vi "nanocal -- nuclear schottky fit -- 2x2 -- V9.vi"() -> ()   [LabVIEW 2021] (continued)
\"Imoff\" -> 0.000000000000   ,  \"στ1\" -> 0.000000000000   ,  \"στS\" -> 0.000000000000   ,  \"στN\" -> 0.000000000000    |>   , \r\"IDS0389_210910_RAW_cal__ref_\" ->   <|    \"ζ\" -> 0.019465629154   ,  \"τ1\" -> 0.035571135590   ,  \"τS\" -> 0.015266533820   ,  \"τN\" -> 0.000260285661   ,  \"τC\" -> 0.004529981538   ,  \"κ0\" -> 0.000000010200   ,  \"mm1\" -> 0.000067219896   ,  \"mm2\" -> 0.019697516293   ,  \"mm3\" -> 0.036165439730   ,  \"T\" -> 1.520000000000   ,  \"B\" -> 8.000000000000   ,  \"θ\" -> 0.000000000000   ,  \"Reoff\" -> -551020.408163265324   ,  \"Imoff\" -> 0.000000000000   ,  \"στ1\" -> 0.011471207658   ,  \"στS\" -> 0.000401132713   ,  \"στN\" -> 0.000048991456    |>   , \r\"IDS0389_210910_RAW_cal__sam_\" ->   <|    \"ζ\" -> 0.011148198813   ,  \"τ1\" -> 0.038849151842   ,  \"τS\" -> 0.019213865355   ,  \"τN\" -> 0.000045035153   ,  \"τC\" -> 0.005536708133   ,  \"κ0\" -> 0.000000011229   ,  \"mm1\" -> 0.000047596165   ,  \"mm2\" -> 0.024836509281   ,  \"mm3\" -> 0.038975357089   ,  \"T\" -> 1.520000000000   ,  \"B\" -> 8.000000000000   ,  \"θ\" -> 0.000000000000   ,  \"Reoff\" -> 0.000000000000   ,  \"Imoff\" -> 0.000000000000   ,  \"στ1\" -> 0.000000000000   ,  \"στS\" -> 0.000000000000   ,  \"στN\" -> 0.000000000000    |>   , \r\"IDS0390_210910_RAW_cal__ref_\" ->   <|    \"ζ\" -> 0.016838578105   ,  \"τ1\" -> 0.032747492196   ,  \"τS\" -> 0.011207679404   ,  \"τN\" -> 0.000117854318   ,  \"τC\" -> 0.003479559601   ,  \"κ0\" -> 0.000000013000   ,  \"mm1\" -> 0.000044274477   ,  \"mm2\" -> 0.014733756508   ,  \"mm3\" -> 0.032965260417   ,  \"T\" -> 1.900000000000   ,  \"B\" -> 8.000000000000   ,  \"θ\" -> 0.000000000000   ,  \"Reoff\" -> -346938.775510204024   ,  \"Imoff\" -> 0.000000000000   ,  \"στ1\" -> 0.005723858997   ,  \"στS\" -> 0.000088565552   ,  \"στN\" -> 0.000007225901    |>   , \r\"IDS0390_210910_RAW_cal__sam_\" ->   <|    \"ζ\" -> 0.010826949430   ,  \"τ1\" -> 0.038768037521   ,  \"τS\" -> 0.012925317198   ,  \"τN\" -> 0.000029157336   ,  \"τC\" -> 0.005196063884   ,  \"κ0\" -> 0.000000013864   ,  \"mm1\" -> 0.000039906108   ,  \"mm2\" -> 0.018195372076   ,  \"mm3\" -> 0.038823555195   ,  \"T\" -> 1.900000000000   ,  \"B\" -> 8.000000000000   ,  \"θ\" -> 0.000000000000   ,  \"Reoff\" -> 0.000000000000   ,  \"Imoff\" -> 0.000000000000   ,  \"στ1\" -> 0.000000000000   ,  \"στS\" -> 0.000000000000   ,  \"στN\" -> 0.000000000000    |>   , \r\"IDS0391_210910_RAW_cal__ref_\" ->   <|    \"ζ\" -> 0.014193901830   ,  \"τ1\" -> 0.092879337404   ,  \"τS\" -> 0.043047307828   ,  \"τN\" -> 0.000265545099   ,  \"τC\" -> 0.003595748456   ,  \"κ0\" -> 0.000000008330   ,  \"mm1\" -> 0.000046539933   ,  \"mm2\" -> 0.046932456699   ,  \"mm3\" -> 0.093423720537   ,  \"T\" -> 1.250000000000   ,  \"B\" -> 8.000000000000   ,  \"θ\" -> 0.000000000000   ,  \"Reoff\" -> -224489.795918366871   ,  \"Imoff\" -> 0.000000000000   ,  \"στ1\" -> 0.004842916086   ,  \"στS\" -> 0.000245036767   ,  \"στN\" -> 0.000003156227    |>   , \r\"IDS0391_210910_RAW_cal__sam_\" ->   <|    \"ζ\" -> 0.010962610928   ,  \"τ1\" -> 0.040398807374   ,  \"τS\" -> 0.051328988590   ,  \"τN\" -> 0.000070281011   ,  \"τC\" -> 0.006422533164   ,  \"κ0\" -> 0.000000008958   ,  \"mm1\" -> 0.000062039854   ,  \"mm2\" -> 0.040240103995   ,  \"mm3\" -> 0.058481936484   ,  \"T\" -> 1.250000000000   ,  \"B\" -> 8.000000000000   ,  \"θ\" -> 0.000000000000   ,  \"Reoff\" -> 0.000000000000   ,  \"Imoff\" -> 0.000000000000   ,  \"στ1\" -> 0.000000000000   ,  \"στS\" -> 0.000000000000   ,  \"στN\" -> 0.000000000000    |>   , \r\"IDS0392_210910_RAW_cal__ref_\" ->   <|    \"ζ\" -> 0.015915665125   ,  \"τ1\" -> 0.061543395288   ,  \"τS\" -> 0.031670398058   ,  \"τN\" -> 0.000248131167   ,  \"τC\" -> 0.003886930831   ,  \"κ0\" -> 0.000000009270   ,  \"mm1\" -> 0.000054412441   ,  \"mm2\" -> 0.035659745539   ,  \"mm3\" -> 0.062142701987   ,  \"T\" -> 1.390000000000   ,  \"B\" -> 8.000000000000   ,  \"θ\" -> 0.000000000000   ,  \"Reoff\" -> -224489.795918366871   ,  \"Imoff\" -> 0.000000000000   ,  \"στ1\" -> 0.005114709163   ,  \"στS\" -> 0.000350050575   ,  \"στN\" -> 0.000004808789    |>   , \r\"IDS0392_210910_RAW_cal__sam_\" ->   <|    \"ζ\" -> 0.010962610928   ,  \"τ1\" -> 0.040398807374   ,  \"τS\" -> 0.051328988590   ,  \"τN\" -> 0.000070281011   ,  \"τC\" -> 0.006422533164   ,  \"κ0\" -> 0.000000008958   ,  \"mm1\" -> 0.000062039854   ,  \"mm2\" -> 0.040240103995   ,  \"mm3\" -> 0.058481936484   ,  \"T\" -> 1.390000000000   ,  \"B\" -> 8.000000000000   ,  \"θ\" -> 0.000000000000   ,  \"Reoff\" -> 0.000000000000   ,  \"Imoff\" -> 0.000000000000   ,  \"στ1\" -> 0.000000000000   ,  \"στS\" -> 0.000000000000   ,  \"στN\" -> 0.000000000000    |>   , \r\"IDS0393_210910_RAW_cal__ref_\" ->   <|    \"ζ\" -> 0.014955256266   ,  \"τ1\" -> 0.026332624911   ,  \"τS\" -> 0.008352670277   ,  \"τN\" -> 0.000164111809   ,  \"τC\" -> 0.002903513034   ,  \"κ0\" -> 0.000000023300   ,  \"mm1\" -> 0.000031957834   ,  \"mm2\" -> 0.011225492804   ,  \"mm3\" -> 0.026622840052   ,  \"T\" -> 3.110000000000   ,  \"B\" -> 8.000000000000   ,  \"θ\" -> 0.000000000000   ,  \"Reoff\" -> -183673.469387754798   ,  \"Imoff\" -> 0.000000000000   ,  \"στ1\" -> 0.001054663608   ,  \"στS\" -> 0.000052081378   ,  \"στN\" -> 0.000002015225    |>   , \r\"IDS0393_210910_RAW_cal__sam_\" ->   <|    \"ζ\" -> 0.010962610928   ,  \"τ1\" -> 0.040398807374   ,  \"τS\" -> 0.051328988590   ,  \"τN\" -> 0.000070281011   ,  \"τC\" -> 0.006422533164   ,  \"κ0\" -> 0.000000008958   ,  \"mm1\" -> 0.000062039854   ,  \"mm2\" -> 0.040240103995   ,  \"mm3\" -> 0.058481936484   ,  \"T\" -> 3.110000000000   ,  \"B\" -> 8.000000000000   ,  \"θ\" -> 0.000000000000   ,  \"Reoff\" -> 0.000000000000   ,  \"Imoff\" -> 0.000000000000   ,  \"στ1\" -> 0.000000000000   ,  \"στS\" -> 0.000000000000   ,  \"στN\" -> 0.000000000000    |>   , \r\"IDS0394_210910_RAW_cal__ref_\" ->   <|    \"ζ\" -> 0.016050939839   ,  \"τ1\" -> 0.020478636674   ,  \"τS\" -> 0.005312059468   ,  \"τN\" -> 0.000195533635   ,  \"τC\" -> 0.002460552068   ,  \"κ0\" -> 0.000000057800   ,  \"mm1\" -> 0.000026789678   ,  \"mm2\" -> 0.007711278862   ,  \"mm3\" -> 0.020797115351   ,  \"T\" -> 5.750000000000   ,  \"B\" -> 8.000000000000   ,  \"θ\" -> 0.000000000000   ,  \"Reoff\" -> -61224.489795917645   ,  \"Imoff\" -> 0.000000000000   ,  \"στ1\" -> 0.004716029121   ,  \"στS\" -> 0.000047047015   ,  \"στN\" -> 0.000018531547    |>   , \r\"IDS0394_210910_RAW_cal__sam_\" ->   <|    \"ζ\" -> 0.010962610928   ,  \"τ1\" -> 0.040398807374   ,  \"τS\" -> 0.051328988590   ,  \"τN\" -> 0.000070281011   ,  \"τC\" -> 0.006422533164   ,  \"κ0\" -> 0.000000008958   ,  \"mm1\" -> 0.000062039854   ,  \"mm2\" -> 0.040240103995   ,  \"mm3\" -> 0.058481936484   ,  \"T\" -> 5.750000000000   ,  \"B\" -> 8.000000000000   ,  \"θ\" -> 0.000000000000   ,  \"Reoff\" -> 0.000000000000   ,  \"Imoff\" -> 0.000000000000   ,  \"στ1\" -> 0.000000000000   ,  \"στS\" -> 0.000000000000   ,  \"στN\" -> 0.000000000000    |>   , \r\"IDS0395_210910_RAW_cal__ref_\" ->   <|    \"ζ\" -> 0.014321636830   ,  \"τ1\" -> 0.097433211743   ,  \"τS\" -> 0.042062236733   ,  \"τN\" -> 0.000244628908   ,  \"τC\" -> 0.003645191846   ,  \"κ0\" -> 0.000000008580   ,  \"mm1\" -> 0.000047465439   ,  \"mm2\" -> 0.046040095215   ,  \"mm3\" -> 0.097903612141   ,  \"T\" -> 1.310000000000   ,  \"B\" -> 8.000000000000   ,  \"θ\" -> 0.000000000000   ,  \"Reoff\" -> -224489.795918366871   ,  \"Imoff\" -> 0.000000000000   ,  \"στ1\" -> 0.012889257014   ,  \"στS\" -> 0.000375170132   ,  \"στN\" -> 0.000004995458    |>   , \r\"IDS0395_210910_RAW_cal__sam_\" ->   <|    \"ζ\" -> 0.010962610928   ,  \"τ1\" -> 0.040398807374   ,  \"τS\" -> 0.051328988590   ,  \"τN\" -> 0.000070281011   ,  \"τC\" -> 0.006422533164   ,  \"κ0\" -> 0.000000008958   ,  \"mm1\" -> 0.000062039854   ,  \"mm2\" -> 0.040240103995   ,  \"mm3\" -> 0.058481936484   ,  \"T\" -> 1.310000000000   ,  \"B\" -> 8.000000000000   ,  \"θ\" -> 0.000000000000   ,  \"Reoff\" -> 0.000000000000   ,  \"Imoff\" -> 0.000000000000   ,  \"στ1\" -> 0.000000000000   ,  \"στS\" -> 0.000000000000   ,  \"στN\" -> 0.000000000000    |>   , \r\"IDS0407_220525_RAW_cal__ref_\" ->   <|    \"ζ\" -> 0.191981162244   ,  \"τ1\" -> 0.000715000000   ,  \"τS\" -> 0.013352458137   ,  \"τN\" -> 0.000004000000   ,  \"τC\" -> 0.002386991901   ,  \"κ0\" -> 0.000000000824   ,  \"mm1\" -> 0.000340641110   ,  \"mm2\" -> 0.000714825522   ,  \"mm3\" -> 0.017967171762   ,  \"T\" -> 0.200000000000   ,  \"B\" -> 0.000000000000   ,  \"θ\" -> 0.000000000000   ,  \"Reoff\" -> 7244897.959183672450   ,  \"Imoff\" -> 0.000000000000   ,  \"στ1\" -> 0.000308977102   ,  \"στS\" -> 0.004347578202   ,  \"στN\" -> 0.000003616273    |>   , \r\"IDS0407_220525_RAW_cal__sam_\" ->   <|    \"ζ\" -> 0.107728168967   ,  \"τ1\" -> 0.019656327090   ,  \"τS\" -> 0.016556579862   ,  \"τN\" -> 0.004758156992   ,  \"τC\" -> 0.001123654800   ,  \"κ0\" -> 0.000000000861   ,  \"mm1\" -> 0.000103510666   ,  \"mm2\" -> 0.011667063931   ,  \"mm3\" -> 0.032620341720   ,  \"T\" -> 0.200000000000   ,  \"B\" -> 0.000000000000   ,  \"θ\" -> 0.000000000000   ,  \"Reoff\" -> -36285714.285714283600   ,  \"Imoff\" -> 0.000000000000   ,  \"στ1\" -> 0.009912643228   ,  \"στS\" -> 0.001520300197   ,  \"στN\" -> 0.002063455636    |>   , \r\"IDS0408_220525_RAW_cal__ref_\" ->   <|    \"ζ\" -> 0.140207229242   ,  \"τ1\" -> 0.000100000000   ,  \"τS\" -> 0.011901792597   ,  \"τN\" -> 0.000001000000   ,  \"τC\" -> 0.001974879987   ,  \"κ0\" -> 0.000000001121   ,  \"mm1\" -> 0.000099990699   ,  \"mm2\" -> 0.000214969707   ,  \"mm3\" -> 0.015331569748   ,  \"T\" -> 0.250000000000   ,  \"B\" -> 0.000000000000   ,  \"θ\" -> 0.000000000000   ,  \"Reoff\" -> 571428.571428570895   ,  \"Imoff\" -> 0.000000000000   ,  \"στ1\" -> 0.000045284114   ,  \"στS\" -> 0.002476603384   ,  \"στN\" -> 0.000000665551    |>   , \r\"IDS0408_220525_RAW_cal__sam_\" ->   <|    \"ζ\" -> 0.086238207773   ,  \"τ1\" -> 0.018354133297   ,  \"τS\" -> 0.015001679768   ,  \"τN\" -> 0.004138272742   ,  \"τC\" -> 0.001377972360   ,  \"κ0\" -> 0.000000001190   ,  \"mm1\" -> 0.000101440698   ,  \"mm2\" -> 0.010941566515   ,  \"mm3\" -> 0.029479646155   ,  \"T\" -> 0.250000000000   ,  \"B\" -> 0.000000000000   ,  \"θ\" -> 0.000000000000   ,  \"Reoff\" -> -26000000.000000000000   ,  \"Imoff\" -> 0.000000000000   ,  \"στ1\" -> 0.004778614510   ,  \"στS\" -> 0.000718856892   ,  \"στN\" -> 0.001132000122    |>   , \r\"IDS0409_220525_RAW_cal__ref_\" ->   <|    \"ζ\" -> 0.126868069995   ,  \"τ1\" -> 0.000131000000   ,  \"τS\" -> 0.010549947054   ,  \"τN\" -> 0.000001000000   ,  \"τC\" -> 0.002473035290   ,  \"κ0\" -> 0.000000001433   ,  \"mm1\" -> 0.000130984950   ,  \"mm2\" -> 0.000234311726   ,  \"mm3\" -> 0.014128263958   ,  \"T\" -> 0.300000000000   ,  \"B\" -> 0.000000000000   ,  \"θ\" -> 0.000000000000   ,  \"Reoff\" -> -408163.265306122600   ,  \"Imoff\" -> 0.000000000000   ,  \"στ1\" -> 0.000026668297   ,  \"στS\" -> 0.002148216121   ,  \"στN\" -> 0.000000592429    |>   , \r\"IDS0409_220525_RAW_cal__sam_\" ->   <|    \"ζ\" -> 0.056561047780   ,  \"τ1\" -> 0.014299678758   ,  \"τS\" -> 0.013769239985   ,  \"τN\" -> 0.003071380883   ,  \"τC\" -> 0.001651608796   ,  \"κ0\" -> 0.000000001520   ,  \"mm1\" -> 0.000079784788   ,  \"mm2\" -> 0.009566648569   ,  \"mm3\" -> 0.024097998227   ,  \"T\" -> 0.300000000000   ,  \"B\" -> 0.000000000000   ,  \"θ\" -> 0.000000000000   ,  \"Reoff\" -> -9836734.693877555430   ,  \"Imoff\" -> 0.000000000000   ,  \"στ1\" -> 0.019869000982   ,  \"στS\" -> 0.002333902836   ,  \"στN\" -> 0.003131938876    |>   , \r\"IDS0410_220525_RAW_cal__ref_\" ->   <|    \"ζ\" -> 0.254310189332   ,  \"τ1\" -> 0.000715000000   ,  \"τS\" -> 0.015590963153   ,  \"τN\" -> 0.000004000000   ,  \"τC\" -> 0.001826387859   ,  \"κ0\" -> 0.000000000621   ,  \"mm1\" -> 0.000344204204   ,  \"mm2\" -> 0.000714835949   ,  \"mm3\" -> 0.021043268891   ,  \"T\" -> 0.170000000000   ,  \"B\" -> 0.000000000000   ,  \"θ\" -> 0.000000000000   ,  \"Reoff\" -> -38967346.938775509600   ,  \"Imoff\" -> 0.000000000000   ,  \"στ1\" -> 0.000454190024   ,  \"στS\" -> 0.005556659278   ,  \"στN\" -> 0.000004239490    |>   , \r\"IDS0410_220525_RAW_cal__sam_\" ->   <|    \"ζ\" -> 0.124885425459   ,  \"τ1\" -> 0.026966294273   ,  \"τS\" -> 0.017799663974   ,  \"τN\" -> 0.005835531331   ,  \"τC\" -> 0.001338388753   ,  \"κ0\" -> 0.000000000710   ,  \"mm1\" -> 0.000140185240   ,  \"mm2\" -> 0.014066781222   ,  \"mm3\" -> 0.040684603290   ,  \"T\" -> 0.170000000000   ,  \"B\" -> 0.000000000000   ,  \"θ\" -> 0.000000000000   ,  \"Reoff\" -> -36285714.285714283600   ,  \"Imoff\" -> 0.000000000000   ,  \"στ1\" -> 0.125291630718   ,  \"στS\" -> 0.008513087182   ,  \"στN\" -> 0.016544280517    |>   , \r\"IDS0411_220525_RAW_cal__ref_\" ->   <|    \"ζ\" -> 0.285546164030   ,  \"τ1\" -> 0.000715000000   ,  \"τS\" -> 0.017341393602   ,  \"τN\" -> 0.000004000000   ,  \"τC\" -> 0.001738862257   ,  \"κ0\" -> 0.000000000531   ,  \"mm1\" -> 0.000363792434   ,  \"mm2\" -> 0.000714850091   ,  \"mm3\" -> 0.023673523941   ,  \"T\" -> 0.150000000000   ,  \"B\" -> 0.000000000000   ,  \"θ\" -> 0.000000000000   ,  \"Reoff\" -> -60000000.000000000000   ,  \"Imoff\" -> 0.000000000000   ,  \"στ1\" -> 0.002198366616   ,  \"στS\" -> 0.030518183124   ,  \"στN\" -> 0.000021250478    |>   , \r\"IDS0411_220525_RAW_cal__sam_\" ->   <|    \"ζ\" -> 0.135609092663   ,  \"τ1\" -> 0.033619209304   ,  \"τS\" -> 0.020242350677   ,  \"τN\" -> 0.009065316224   ,  \"τC\" -> 0.001338388753   ,  \"κ0\" -> 0.000000000610   ,  \"mm1\" -> 0.000151964902   ,  \"mm2\" -> 0.015437467353   ,  \"mm3\" -> 0.052650218819   ,  \"T\" -> 0.150000000000   ,  \"B\" -> 0.000000000000   ,  \"θ\" -> 0.000000000000   ,  \"Reoff\" -> -36285714.285714283600   ,  \"Imoff\" -> 0.000000000000   ,  \"στ1\" -> 0.012006153279   ,  \"στS\" -> 0.002506054906   ,  \"στN\" -> 0.002275285607    |>   , \r\"IDS0412_220525_RAW_cal__ref_\" ->   <|    \"ζ\" -> 0.335616597388   ,  \"τ1\" -> 0.000100000000   ,  \"τS\" -> 0.019397772519   ,  \"τN\" -> 0.000001000000   ,  \"τC\" -> 0.001855570949   ,  \"κ0\" -> 0.000000000419   ,  \"mm1\" -> 0.000099994748   ,  \"mm2\" -> 0.000442151707   ,  \"mm3\" -> 0.027322747041   ,  \"T\" -> 0.120000000000   ,  \"B\" -> 0.000000000000   ,  \"θ\" -> 0.000000000000   ,  \"Reoff\" -> -114641566.265060246000   ,  \"Imoff\" -> 0.000000000000   ,  \"στ1\" -> 0.000060137518   ,  \"στS\" -> 0.005391505874   ,  \"στN\" -> 0.000000931452    |>   , \r\"IDS0412_220525_RAW_cal__sam_\" ->   <|    \"ζ\" -> 0.141872667412   ,  \"τ1\" -> 0.045522682755   ,  \"τS\" -> 0.024683404671   ,  \"τN\" -> 0.014187266741   ,  \"τC\" -> 0.001029575567   ,  \"κ0\" -> 0.000000000485   ,  \"mm1\" -> 0.000123931838   ,  \"mm2\" -> 0.018251391889   ,  \"mm3\" -> 0.072562291843   ,  \"T\" -> 0.120000000000   ,  \"B\" -> 0.000000000000   ,  \"θ\" -> 0.000000000000   ,  \"Reoff\" -> -36285714.285714283600   ,  \"Imoff\" -> 0.000000000000   ,  \"στ1\" -> 0.019575103663   ,  \"στS\" -> 0.006297786999   ,  \"στN\" -> 0.007663344539    |>   , \r\"IDS0413_220525_RAW_cal__ref_\" ->   <|    \"ζ\" -> 0.101522362019   ,  \"τ1\" -> 0.000131000000   ,  \"τS\" -> 0.009935467589   ,  \"τN\" -> 0.000001000000   ,  \"τC\" -> 0.002817089686   ,  \"κ0\" -> 0.000000001826   ,  \"mm1\" -> 0.000130982425   ,  \"mm2\" -> 0.000209693311   ,  \"mm3\" -> 0.013552655199   ,  \"T\" -> 0.360000000000   ,  \"B\" -> 0.000000000000   ,  \"θ\" -> 0.000000000000   ,  \"Reoff\" -> -346938.775510204024   ,  \"Imoff\" -> 0.000000000000   ,  \"στ1\" -> 0.000056432011   ,  \"στS\" -> 0.002135806697   ,  \"στN\" -> 0.000000647721    |>   , \r\"IDS0413_220525_RAW_cal__sam_\" ->   <|    \"ζ\" -> 0.044690907244   ,  \"τ1\" -> 0.013320614253   ,  \"τS\" -> 0.013760942515   ,  \"τN\" -> 0.002327045716   ,  \"τC\" -> 0.001523256988   ,  \"κ0\" -> 0.000000001960   ,  \"mm1\" -> 0.000059136229   ,  \"mm2\" -> 0.009591413737   ,  \"mm3\" -> 0.022000296296   ,  \"T\" -> 0.360000000000   ,  \"B\" -> 0.000000000000   ,  \"θ\" -> 0.000000000000   ,  \"Reoff\" -> -7142857.142857141800   ,  \"Imoff\" -> 0.000000000000   ,  \"στ1\" -> 0.002601583253   ,  \"στS\" -> 0.000378567326   ,  \"στN\" -> 0.000355149378    |>   , \r\"IDS0414_220525_RAW_cal__ref_\" ->   <|    \"ζ\" -> 0.086864800991   ,  \"τ1\" -> 0.000131000000   ,  \"τS\" -> 0.009397396069   ,  \"τN\" -> 0.000001000000   ,  \"τC\" -> 0.003391459878   ,  \"κ0\" -> 0.000000002303   ,  \"mm1\" -> 0.000130980131   ,  \"mm2\" -> 0.000206638483   ,  \"mm3\" -> 0.013399627137   ,  \"T\" -> 0.430000000000   ,  \"B\" -> 0.000000000000   ,  \"θ\" -> 0.000000000000   ,  \"Reoff\" -> -163265.306122449226   ,  \"Imoff\" -> 0.000000000000   ,  \"στ1\" -> 0.000060821776   ,  \"στS\" -> 0.002038590742   ,  \"στN\" -> 0.000000647790    |>   , \r\"IDS0414_220525_RAW_cal__sam_\" ->   <|    \"ζ\" -> 0.036206503728   ,  \"τ1\" -> 0.010323598347   ,  \"τS\" -> 0.013793333734   ,  \"τN\" -> 0.001947462554   ,  \"τC\" -> 0.001576858934   ,  \"κ0\" -> 0.000000002450   ,  \"mm1\" -> 0.000049775806   ,  \"mm2\" -> 0.008169881573   ,  \"mm3\" -> 0.019991515390   ,  \"T\" -> 0.430000000000   ,  \"B\" -> 0.000000000000   ,  \"θ\" -> 0.000000000000   ,  \"Reoff\" -> -5183673.469387754800   ,  \"Imoff\" -> 0.000000000000   ,  \"στ1\" -> 0.000547128250   ,  \"στS\" -> 0.000218959699   ,  \"στN\" -> 0.000102085685    |>   , \r\"IDS0415_220525_RAW_cal__ref_\" ->   <|    \"ζ\" -> 0.068474978829   ,  \"τ1\" -> 0.000131000000   ,  \"τS\" -> 0.009236829500   ,  \"τN\" -> 0.000001000000   ,  \"τC\" -> 0.004057709809   ,  \"κ0\" -> 0.000000002964   ,  \"mm1\" -> 0.000130976218   ,  \"mm2\" -> 0.000186804029   ,  \"mm3\" -> 0.013741319241   ,  \"T\" -> 0.530000000000   ,  \"B\" -> 0.000000000000   ,  \"θ\" -> 0.000000000000   ,  \"Reoff\" -> 20408.163265305571   ,  \"Imoff\" -> 0.000000000000   ,  \"στ1\" -> 0.000060728643   ,  \"στS\" -> 0.002214555558   ,  \"στN\" -> 0.000000706219    |>   , \r\"IDS0415_220525_RAW_cal__sam_\" ->   <|    \"ζ\" -> 0.029049723552   ,  \"τ1\" -> 0.007716049820   ,  \"τS\" -> 0.014447051972   ,  \"τN\" -> 0.001246053989   ,  \"τC\" -> 0.001554051920   ,  \"κ0\" -> 0.000000003200   ,  \"mm1\" -> 0.000039813384   ,  \"mm2\" -> 0.006805314073   ,  \"mm3\" -> 0.018573960634   ,  \"T\" -> 0.530000000000   ,  \"B\" -> 0.000000000000   ,  \"θ\" -> 0.000000000000   ,  \"Reoff\" -> -3959183.673469387000   ,  \"Imoff\" -> 0.000000000000   ,  \"στ1\" -> 0.000764801064   ,  \"στS\" -> 0.002293201092   ,  \"στN\" -> 0.000221114317    |>   , \r\"IDS0416_220525_RAW_cal__ref_\" ->   <|    \"ζ\" -> 0.054673110609   ,  \"τ1\" -> 0.000131000000   ,  \"τS\" -> 0.009614471187   ,  \"τN\" -> 0.000001000000   ,  \"τC\" -> 0.004596429242   ,  \"κ0\" -> 0.000000003616   ,  \"mm1\" -> 0.000130970546   ,  \"mm2\" -> 0.000165845795   ,  \"mm3\" -> 0.014571791808   ,  \"T\" -> 0.630000000000   ,  \"B\" -> 0.000000000000   ,  \"θ\" -> 0.000000000000   ,  \"Reoff\" -> -40816.326530612074   ,  \"Imoff\" -> 0.000000000000   ,  \"στ1\" -> 0.000081473849   ,  \"στS\" -> 0.003083885003   ,  \"στN\" -> 0.000000972224    |>   , \r\"IDS0416_220525_RAW_cal__sam_\" ->   <|    \"ζ\" -> 0.022998692784   ,  \"τ1\" -> 0.007393021158   ,  \"τS\" -> 0.015620230500   ,  \"τN\" -> 0.001040733682   ,  \"τC\" -> 0.001765774011   ,  \"κ0\" -> 0.000000003911   ,  \"mm1\" -> 0.000035818495   ,  \"mm2\" -> 0.006739334009   ,  \"mm3\" -> 0.019427787243   ,  \"T\" -> 0.630000000000   ,  \"B\" -> 0.000000000000   ,  \"θ\" -> 0.000000000000   ,  \"Reoff\" -> -2408163.265306121670   ,  \"Imoff\" -> 0.000000000000   ,  \"στ1\" -> 0.000980763421   ,  \"στS\" -> 0.002016923628   ,  \"στN\" -> 0.000219391445    |>   , \r\"IDS0417_220525_RAW_cal__ref_\" ->   <|    \"ζ\" -> 0.032259473500   ,  \"τ1\" -> 0.000131000000   ,  \"τS\" -> 0.013853650648   ,  \"τN\" -> 0.000001000000   ,  \"τC\" -> 0.003329884920   ,  \"κ0\" -> 0.000000004970   ,  \"mm1\" -> 0.000084814686   ,  \"mm2\" -> 0.000130995471   ,  \"mm3\" -> 0.017546669145   ,  \"T\" -> 0.830000000000   ,  \"B\" -> 0.000000000000   ,  \"θ\" -> 0.000000000000   ,  \"Reoff\" -> -959183.673469387924   ,  \"Imoff\" -> 0.000000000000   ,  \"στ1\" -> 0.000056019641   ,  \"στS\" -> 0.002791706038   ,  \"στN\" -> 0.000000650322    |>   , \r\"IDS0417_220525_RAW_cal__sam_\" ->   <|    \"ζ\" -> 0.020422056832   ,  \"τ1\" -> 0.006457484957   ,  \"τS\" -> 0.019722165301   ,  \"τN\" -> 0.000729413719   ,  \"τC\" -> 0.001622930071   ,  \"κ0\" -> 0.000000005380   ,  \"mm1\" -> 0.000030097695   ,  \"mm2\" -> 0.006162713408   ,  \"mm3\" -> 0.022756846254   ,  \"T\" -> 0.830000000000   ,  \"B\" -> 0.000000000000   ,  \"θ\" -> 0.000000000000   ,  \"Reoff\" -> -2081632.653061224150   ,  \"Imoff\" -> 0.000000000000   ,  \"στ1\" -> 0.000977899540   ,  \"στS\" -> 0.002370947727   ,  \"στN\" -> 0.000160479256    |>   , \r\"IDS0418_220525_RAW_cal__ref_\" ->   <|    \"ζ\" -> 0.101578237405   ,  \"τ1\" -> 0.000131000000   ,  \"τS\" -> 0.019496503151   ,  \"τN\" -> 0.000001000000   ,  \"τC\" -> 0.002824938622   ,  \"κ0\" -> 0.000000006490   ,  \"mm1\" -> 0.000130992305   ,  \"mm2\" -> 0.000232437503   ,  \"mm3\" -> 0.024070533970   ,  \"T\" -> 1.120000000000   ,  \"B\" -> 0.000000000000   ,  \"θ\" -> 0.000000000000   ,  \"Reoff\" -> -9469387.755102038390   ,  \"Imoff\" -> 0.000000000000   ,  \"στ1\" -> 0.000013096925   ,  \"στS\" -> 0.001629413974   ,  \"στN\" -> 0.000000279483    |>   , \r\"IDS0418_220525_RAW_cal__sam_\" ->   <|    \"ζ\" -> 0.010833914814   ,  \"τ1\" -> 0.006105280968   ,  \"τS\" -> 0.027771405990   ,  \"τN\" -> 0.000655710517   ,  \"τC\" -> 0.001898693697   ,  \"κ0\" -> 0.000000007420   ,  \"mm1\" -> 0.000019072683   ,  \"mm2\" -> 0.005941306089   ,  \"mm3\" -> 0.030778689359   ,  \"T\" -> 1.120000000000   ,  \"B\" -> 0.000000000000   ,  \"θ\" -> 0.000000000000   ,  \"Reoff\" -> -608163.265306122367   ,  \"Imoff\" -> 0.000000000000   ,  \"στ1\" -> 0.001326459237   ,  \"στS\" -> 0.003728359065   ,  \"στN\" -> 0.000181682896    |>   , \r\"IDS0419_220525_RAW_cal__ref_\" ->   <|    \"ζ\" -> 0.054328127598   ,  \"τ1\" -> 0.000131000000   ,  \"τS\" -> 0.041800630964   ,  \"τN\" -> 0.000001000000   ,  \"τC\" -> 0.008136787294   ,  \"κ0\" -> 0.000000011908   ,  \"mm1\" -> 0.000130996584   ,  \"mm2\" -> 0.000356366999   ,  \"mm3\" -> 0.051853059016   ,  \"T\" -> 1.900000000000   ,  \"B\" -> 0.000000000000   ,  \"θ\" -> 0.000000000000   ,  \"Reoff\" -> -2412244.897959183900   ,  \"Imoff\" -> 0.000000000000   ,  \"στ1\" -> 0.000075606348   ,  \"στS\" -> 0.006052354245   ,  \"στN\" -> 0.000000670558    |>   , \r\"IDS0419_220525_RAW_cal__sam_\" ->   <|    \"ζ\" -> 0.011595776290   ,  \"τ1\" -> 0.006117918264   ,  \"τS\" -> 0.061916055974   ,  \"τN\" -> 0.000669101537   ,  \"τC\" -> 0.002022450323   ,  \"κ0\" -> 0.000000012950   ,  \"mm1\" -> 0.000022465670   ,  \"mm2\" -> 0.006048051710   ,  \"mm3\" -> 0.065380732203   ,  \"T\" -> 1.900000000000   ,  \"B\" -> 0.000000000000   ,  \"θ\" -> 0.000000000000   ,  \"Reoff\" -> -608163.265306122367   ,  \"Imoff\" -> 0.000000000000   ,  \"στ1\" -> 0.001547930555   ,  \"στS\" -> 0.007827805463   ,  \"στN\" -> 0.000227173092    |>   , \r\"IDS0420_220525_RAW_cal__ref_\" ->   <|    \"ζ\" -> 0.054690281764   ,  \"τ1\" -> 0.000131000000   ,  \"τS\" -> 0.045992171451   ,  \"τN\" -> 0.000001000000   ,  \"τC\" -> 0.007372108350   ,  \"κ0\" -> 0.000000013567   ,  \"mm1\" -> 0.000130996911   ,  \"mm2\" -> 0.000333838788   ,  \"mm3\" -> 0.055546823607   ,  \"T\" -> 2.100000000000   ,  \"B\" -> 0.000000000000   ,  \"θ\" -> 0.000000000000   ,  \"Reoff\" -> -2412244.897959183900   ,  \"Imoff\" -> 0.000000000000   ,  \"στ1\" -> 0.000040532955   ,  \"στS\" -> 0.006090399823   ,  \"στN\" -> 0.000000564115    |>   , \r\"IDS0420_220525_RAW_cal__sam_\" ->   <|    \"ζ\" -> 0.011850996022   ,  \"τ1\" -> 0.005764384736   ,  \"τS\" -> 0.066220067505   ,  \"τN\" -> 0.000645440877   ,  \"τC\" -> 0.002901198812   ,  \"κ0\" -> 0.000000014700   ,  \"mm1\" -> 0.000032584327   ,  \"mm2\" -> 0.005706320364   ,  \"mm3\" -> 0.070584610113   ,  \"T\" -> 2.100000000000   ,  \"B\" -> 0.000000000000   ,  \"θ\" -> 0.000000000000   ,  \"Reoff\" -> -461224.489795918343   ,  \"Imoff\" -> 0.000000000000   ,  \"στ1\" -> 0.000879947943   ,  \"στS\" -> 0.005816006372   ,  \"στN\" -> 0.000150645668    |>   , \r\"IDS0421_220525_RAW_cal__ref_\" ->   <|    \"ζ\" -> 0.060508336123   ,  \"τ1\" -> 0.000131000000   ,  \"τS\" -> 0.007131357442   ,  \"τN\" -> 0.000001000000   ,  \"τC\" -> 0.009850008228   ,  \"κ0\" -> 0.000000015720   ,  \"mm1\" -> 0.000130969869   ,  \"mm2\" -> 0.000247654950   ,  \"mm3\" -> 0.017166307932   ,  \"T\" -> 2.300000000000   ,  \"B\" -> 0.000000000000   ,  \"θ\" -> 0.000000000000   ,  \"Reoff\" -> -391836.734693877398   ,  \"Imoff\" -> 0.000000000000   ,  \"στ1\" -> 0.000074085946   ,  \"στS\" -> 0.002081131924   ,  \"στN\" -> 0.000000819648    |>   , \r\"IDS0421_220525_RAW_cal__sam_\" ->   <|    \"ζ\" -> 0.017472306497   ,  \"τ1\" -> 0.005884707777   ,  \"τS\" -> 0.018273540555   ,  \"τN\" -> 0.000393530305   ,  \"τC\" -> 0.002873982576   ,  \"κ0\" -> 0.000000016000   ,  \"mm1\" -> 0.000042829990   ,  \"mm2\" -> 0.005738391469   ,  \"mm3\" -> 0.021970696537   ,  \"T\" -> 2.300000000000   ,  \"B\" -> 0.000000000000   ,  \"θ\" -> 0.000000000000   ,  \"Reoff\" -> -616326.530612244968   ,  \"Imoff\" -> 0.000000000000   ,  \"στ1\" -> 0.001449504442   ,  \"στS\" -> 0.003094967894   ,  \"στN\" -> 0.000132016087    |>   , \r\"IDS0422_220525_RAW_cal__ref_\" ->   <|    \"ζ\" -> 0.065958272689   ,  \"τ1\" -> 0.000131000000   ,  \"τS\" -> 0.004874385482   ,  \"τN\" -> 0.000001000000   ,  \"τC\" -> 0.006474262429   ,  \"κ0\" -> 0.000000022464   ,  \"mm1\" -> 0.000130934041   ,  \"mm2\" -> 0.000181249477   ,  \"mm3\" -> 0.011490036398   ,  \"T\" -> 3.100000000000   ,  \"B\" -> 0.000000000000   ,  \"θ\" -> 0.000000000000   ,  \"Reoff\" -> -391836.734693877398   ,  \"Imoff\" -> 0.000000000000   ,  \"στ1\" -> 0.000042174931   ,  \"στS\" -> 0.000833454188   ,  \"στN\" -> 0.000000451005    |>   , \r\"IDS0422_220525_RAW_cal__sam_\" ->   <|    \"ζ\" -> 0.013782660001   ,  \"τ1\" -> 0.005602489845   ,  \"τS\" -> 0.011122141420   ,  \"τN\" -> 0.000341635093   ,  \"τC\" -> 0.002887063483   ,  \"κ0\" -> 0.000000023500   ,  \"mm1\" -> 0.000031317292   ,  \"mm2\" -> 0.005389288482   ,  \"mm3\" -> 0.014690725401   ,  \"T\" -> 3.100000000000   ,  \"B\" -> 0.000000000000   ,  \"θ\" -> 0.000000000000   ,  \"Reoff\" -> -338775.510204081656   ,  \"Imoff\" -> 0.000000000000   ,  \"στ1\" -> 0.000787586702   ,  \"στS\" -> 0.001319427978   ,  \"στN\" -> 0.000072408344    |>   , \r\"IDS0424_220526_RAW_cal__ref_\" ->   <|    \"ζ\" -> 0.257865003377   ,  \"τ1\" -> 0.052975439100   ,  \"τS\" -> 0.072879585760   ,  \"τN\" -> 0.046129702285   ,  \"τC\" -> 0.000850997737   ,  \"κ0\" -> 0.000000000770   ,  \"mm1\" -> 0.000173173247   ,  \"mm2\" -> 0.027881728109   ,  \"mm3\" -> 0.175469153990   ,  \"T\" -> 0.190000000000   ,  \"B\" -> 10.000000000000   ,  \"θ\" -> 0.000000000000   ,  \"Reoff\" -> -49000000.000000000000   ,  \"Imoff\" -> 0.000000000000   ,  \"στ1\" -> 0.038419382366   ,  \"στS\" -> 0.010252018344   ,  \"στN\" -> 0.015460977129    |>   , \r\"IDS0424_220526_RAW_cal__sam_\" ->   <|    \"ζ\" -> 0.143096873941   ,  \"τ1\" -> 0.119527741552   ,  \"τS\" -> 0.213771204505   ,  \"τN\" -> 0.133065206622   ,  \"τC\" -> 0.001041786526   ,  \"κ0\" -> 0.000000000890   ,  \"mm1\" -> 0.000129929317   ,  \"mm2\" -> 0.064852834373   ,  \"mm3\" -> 0.452054381716   ,  \"T\" -> 0.190000000000   ,  \"B\" -> 10.000000000000   ,  \"θ\" -> 0.000000000000   ,  \"Reoff\" -> -41461224.489795915800   ,  \"Imoff\" -> 0.000000000000   ,  \"στ1\" -> 0.142328196867   ,  \"στS\" -> 0.153709890516   ,  \"στN\" -> 0.034979737706    |>   , \r\"IDS0425_220526_RAW_cal__ref_\" ->   <|    \"ζ\" -> 0.150640974704   ,  \"τ1\" -> 0.034197272609   ,  \"τS\" -> 0.049670713863   ,  \"τN\" -> 0.019296596370   ,  \"τC\" -> 0.000986151726   ,  \"κ0\" -> 0.000000001118   ,  \"mm1\" -> 0.000127191823   ,  \"mm2\" -> 0.021308290346   ,  \"mm3\" -> 0.093104555235   ,  \"T\" -> 0.250000000000   ,  \"B\" -> 10.000000000000   ,  \"θ\" -> 0.000000000000   ,  \"Reoff\" -> -20330612.244897961600   ,  \"Imoff\" -> 0.000000000000   ,  \"στ1\" -> 0.016426599332   ,  \"στS\" -> 0.002938321228   ,  \"στN\" -> 0.003825151273    |>   , \r\"IDS0425_220526_RAW_cal__sam_\" ->   <|    \"ζ\" -> 0.080613368975   ,  \"τ1\" -> 0.039981630615   ,  \"τS\" -> 0.067451052819   ,  \"τN\" -> 0.024952731947   ,  \"τC\" -> 0.001301901326   ,  \"κ0\" -> 0.000000001270   ,  \"mm1\" -> 0.000095538727   ,  \"mm2\" -> 0.025680137218   ,  \"mm3\" -> 0.115360621158   ,  \"T\" -> 0.250000000000   ,  \"B\" -> 10.000000000000   ,  \"θ\" -> 0.000000000000   ,  \"Reoff\" -> -15077551.020408168400   ,  \"Imoff\" -> 0.000000000000   ,  \"στ1\" -> 0.017921325903   ,  \"στS\" -> 0.008554959302   ,  \"στN\" -> 0.012696106226    |>   , \r\"IDS0426_220526_RAW_cal__ref_\" ->   <|    \"ζ\" -> 0.110651122840   ,  \"τ1\" -> 0.023688979566   ,  \"τS\" -> 0.041888104291   ,  \"τN\" -> 0.009400965947   ,  \"τC\" -> 0.001054144270   ,  \"κ0\" -> 0.000000001430   ,  \"mm1\" -> 0.000102915193   ,  \"mm2\" -> 0.017560405745   ,  \"mm3\" -> 0.064044066348   ,  \"T\" -> 0.300000000000   ,  \"B\" -> 10.000000000000   ,  \"θ\" -> 0.000000000000   ,  \"Reoff\" -> -13408163.265306122600   ,  \"Imoff\" -> 0.000000000000   ,  \"στ1\" -> 0.009988334429   ,  \"στS\" -> 0.001537868285   ,  \"στN\" -> 0.001719296338    |>   , \r\"IDS0426_220526_RAW_cal__sam_\" ->   <|    \"ζ\" -> 0.000000000000   ,  \"τ1\" -> 0.000000000000   ,  \"τS\" -> 0.000000000000   ,  \"τN\" -> 0.000000000000   ,  \"τC\" -> 0.000000000000   ,  \"κ0\" -> 0.000000000000   ,  \"mm1\" -> 0.000000000000   ,  \"mm2\" -> 0.000000000000   ,  \"mm3\" -> 0.000000000000   ,  \"T\" -> 0.300000000000   ,  \"B\" -> 10.000000000000   ,  \"θ\" -> 0.000000000000   ,  \"Reoff\" -> 0.000000000000   ,  \"Imoff\" -> 0.000000000000   ,  \"στ1\" -> 0.000000000000   ,  \"στS\" -> 0.000000000000   ,  \"στN\" -> 0.000000000000    |>   , \r\"IDS0427_220526_RAW_cal__ref_\" ->   <|    \"ζ\" -> 0.400378368532   ,  \"τ1\" -> 0.070020543839   ,  \"τS\" -> 0.131128875469   ,  \"τN\" -> 0.110503953528   ,  \"τC\" -> 0.000929381263   ,  \"κ0\" -> 0.000000000547   ,  \"mm1\" -> 0.000264755544   ,  \"mm2\" -> 0.034447529222   ,  \"mm3\" -> 0.374615027191   ,  \"T\" -> 0.150000000000   ,  \"B\" -> 10.000000000000   ,  \"θ\" -> 0.000000000000   ,  \"Reoff\" -> -90065306.122448980800   ,  \"Imoff\" -> 0.000000000000   ,  \"στ1\" -> 0.115545840550   ,  \"στS\" -> 0.062145974598   ,  \"στN\" -> 0.087083233243    |>   , \r\"IDS0427_220526_RAW_cal__sam_\" ->   <|    \"ζ\" -> 0.000000000000   ,  \"τ1\" -> 0.000000000000   ,  \"τS\" -> 0.000000000000   ,  \"τN\" -> 0.000000000000   ,  \"τC\" -> 0.000000000000   ,  \"κ0\" -> 0.000000000000   ,  \"mm1\" -> 0.000000000000   ,  \"mm2\" -> 0.000000000000   ,  \"mm3\" -> 0.000000000000   ,  \"T\" -> 0.150000000000   ,  \"B\" -> 10.000000000000   ,  \"θ\" -> 0.000000000000   ,  \"Reoff\" -> 0.000000000000   ,  \"Imoff\" -> 0.000000000000   ,  \"στ1\" -> 0.000000000000   ,  \"στS\" -> 0.000000000000   ,  \"στN\" -> 0.000000000000    |>   , \r\"IDS0428_220526_RAW_cal__ref_\" ->   <|    \"ζ\" -> 0.082438962756   ,  \"τ1\" -> 0.024345135189   ,  \"τS\" -> 0.039010983719   ,  \"τN\" -> 0.005604008996   ,  \"τC\" -> 0.001011795266   ,  \"κ0\" -> 0.000000001850   ,  \"mm1\" -> 0.000075386231   ,  \"mm2\" -> 0.019395489677   ,  \"mm3\" -> 0.054179060985   ,  \"T\" -> 0.360000000000   ,  \"B\" -> 10.000000000000   ,  \"θ\" -> 0.000000000000   ,  \"Reoff\" -> -9632653.061224490410   ,  \"Imoff\" -> 0.000000000000   ,  \"στ1\" -> 0.001903743103   ,  \"στS\" -> 0.000574153374   ,  \"στN\" -> 0.002568840036    |>   , \r\"IDS0428_220526_RAW_cal__sam_\" ->   <|    \"ζ\" -> 0.000000000000   ,  \"τ1\" -> 0.000000000000   ,  \"τS\" -> 0.000000000000   ,  \"τN\" -> 0.000000000000   ,  \"τC\" -> 0.000000000000   ,  \"κ0\" -> 0.000000000000   ,  \"mm1\" -> 0.000000000000   ,  \"mm2\" -> 0.000000000000   ,  \"mm3\" -> 0.000000000000   ,  \"T\" -> 0.360000000000   ,  \"B\" -> 10.000000000000   ,  \"θ\" -> 0.000000000000   ,  \"Reoff\" -> 0.000000000000   ,  \"Imoff\" -> 0.000000000000   ,  \"στ1\" -> 0.000000000000   ,  \"στS\" -> 0.000000000000   ,  \"στN\" -> 0.000000000000    |>   , \r\"IDS0429_220526_RAW_cal__ref_\" ->   <|    \"ζ\" -> 0.070312011413   ,  \"τ1\" -> 0.022685637424   ,  \"τS\" -> 0.038017817435   ,  \"τN\" -> 0.003686111033   ,  \"τC\" -> 0.000858092615   ,  \"κ0\" -> 0.000000002230   ,  \"mm1\" -> 0.000055279779   ,  \"mm2\" -> 0.019266175315   ,  \"mm3\" -> 0.048858490507   ,  \"T\" -> 0.420000000000   ,  \"B\" -> 10.000000000000   ,  \"θ\" -> 0.000000000000   ,  \"Reoff\" -> -9632653.061224490410   ,  \"Imoff\" -> 0.000000000000   ,  \"στ1\" -> 0.001355990341   ,  \"στS\" -> 0.000271524957   ,  \"στN\" -> 0.000140246830    |>   , \r\"IDS0429_220526_RAW_cal__sam_\" ->   <|    \"ζ\" -> 0.000000000000   ,  \"τ1\" -> 0.000000000000   ,  \"τS\" -> 0.000000000000   ,  \"τN\" -> 0.000000000000   ,  \"τC\" -> 0.000000000000   ,  \"κ0\" -> 0.000000000000   ,  \"mm1\" -> 0.000000000000   ,  \"mm2\" -> 0.000000000000   ,  \"mm3\" -> 0.000000000000   ,  \"T\" -> 0.420000000000   ,  \"B\" -> 10.000000000000   ,  \"θ\" -> 0.000000000000   ,  \"Reoff\" -> 0.000000000000   ,  \"Imoff\" -> 0.000000000000   ,  \"στ1\" -> 0.000000000000   ,  \"στS\" -> 0.000000000000   ,  \"στN\" -> 0.000000000000    |>   , \r\"IDS0430_220526_RAW_cal__ref_\" ->   <|    \"ζ\" -> 0.045461152604   ,  \"τ1\" -> 0.022205538452   ,  \"τS\" -> 0.038393095410   ,  \"τN\" -> 0.002129809404   ,  \"τC\" -> 0.001500655488   ,  \"κ0\" -> 0.000000002910   ,  \"mm1\" -> 0.000062998174   ,  \"mm2\" -> 0.020118168551   ,  \"mm3\" -> 0.045890149989   ,  \"T\" -> 0.520000000000   ,  \"B\" -> 10.000000000000   ,  \"θ\" -> 0.000000000000   ,  \"Reoff\" -> -3224489.795918375260   ,  \"Imoff\" -> 0.000000000000   ,  \"στ1\" -> 0.001544196925   ,  \"στS\" -> 0.000197668706   ,  \"στN\" -> 0.000070756968    |>   , \r\"IDS0430_220526_RAW_cal__sam_\" ->   <|    \"ζ\" -> 0.000000000000   ,  \"τ1\" -> 0.000000000000   ,  \"τS\" -> 0.000000000000   ,  \"τN\" -> 0.000000000000   ,  \"τC\" -> 0.000000000000   ,  \"κ0\" -> 0.000000000000   ,  \"mm1\" -> 0.000000000000   ,  \"mm2\" -> 0.000000000000   ,  \"mm3\" -> 0.000000000000   ,  \"T\" -> 0.520000000000   ,  \"B\" -> 10.000000000000   ,  \"θ\" -> 0.000000000000   ,  \"Reoff\" -> 0.000000000000   ,  \"Imoff\" -> 0.000000000000   ,  \"στ1\" -> 0.000000000000   ,  \"στS\" -> 0.000000000000   ,  \"στN\" -> 0.000000000000    |>   , \r\"IDS0431_220527_RAW_cal__ref_\" ->   <|    \"ζ\" -> 0.560959524386   ,  \"τ1\" -> 0.162135875123   ,  \"τS\" -> 0.311559023690   ,  \"τN\" -> 0.235565493895   ,  \"τC\" -> 0.000943331482   ,  \"κ0\" -> 0.000000000415   ,  \"mm1\" -> 0.000338581832   ,  \"mm2\" -> 0.084703245290   ,  \"mm3\" -> 0.932076606233   ,  \"T\" -> 0.120000000000   ,  \"B\" -> 10.000000000000   ,  \"θ\" -> 0.000000000000   ,  \"Reoff\" -> -130387755.102040812000   ,  \"Imoff\" -> 0.000000000000   ,  \"στ1\" -> 0.196821258023   ,  \"στS\" -> 0.124985342591   ,  \"στN\" -> 0.122755892139    |>   , \r\"IDS0431_220527_RAW_cal__sam_\" ->   <|    \"ζ\" -> 0.000000000000   ,  \"τ1\" -> 0.000000000000   ,  \"τS\" -> 0.000000000000   ,  \"τN\" -> 0.000000000000   ,  \"τC\" -> 0.000000000000   ,  \"κ0\" -> 0.000000000000   ,  \"mm1\" -> 0.000000000000   ,  \"mm2\" -> 0.000000000000   ,  \"mm3\" -> 0.000000000000   ,  \"T\" -> 0.120000000000   ,  \"B\" -> 10.000000000000   ,  \"θ\" -> 0.000000000000   ,  \"Reoff\" -> 0.000000000000   ,  \"Imoff\" -> 0.000000000000   ,  \"στ1\" -> 0.000000000000   ,  \"στS\" -> 0.000000000000   ,  \"στN\" -> 0.000000000000    |>   , \r\"IDS0432_220527_RAW_cal__ref_\" ->   <|    \"ζ\" -> 0.302881771202   ,  \"τ1\" -> 0.053970650610   ,  \"τS\" -> 0.084832458604   ,  \"τN\" -> 0.070036651320   ,  \"τC\" -> 0.000864371133   ,  \"κ0\" -> 0.000000000675   ,  \"mm1\" -> 0.000199736141   ,  \"mm2\" -> 0.026051282095   ,  \"mm3\" -> 0.230360143749   ,  \"T\" -> 0.170000000000   ,  \"B\" -> 10.000000000000   ,  \"θ\" -> 0.000000000000   ,  \"Reoff\" -> -65714285.714285716400   ,  \"Imoff\" -> 0.000000000000   ,  \"στ1\" -> 0.042116863127   ,  \"στS\" -> 0.016985307293   ,  \"στN\" -> 0.023565277591    |>   , \r\"IDS0432_220527_RAW_cal__sam_\" ->   <|    \"ζ\" -> 0.000000000000   ,  \"τ1\" -> 0.000000000000   ,  \"τS\" -> 0.000000000000   ,  \"τN\" -> 0.000000000000   ,  \"τC\" -> 0.000000000000   ,  \"κ0\" -> 0.000000000000   ,  \"mm1\" -> 0.000000000000   ,  \"mm2\" -> 0.000000000000   ,  \"mm3\" -> 0.000000000000   ,  \"T\" -> 0.170000000000   ,  \"B\" -> 10.000000000000   ,  \"θ\" -> 0.000000000000   ,  \"Reoff\" -> 0.000000000000   ,  \"Imoff\" -> 0.000000000000   ,  \"στ1\" -> 0.000000000000   ,  \"στS\" -> 0.000000000000   ,  \"στN\" -> 0.000000000000    |>   , \r\"IDS0433_220527_RAW_cal__ref_\" ->   <|    \"ζ\" -> 0.035999178559   ,  \"τ1\" -> 0.021236822586   ,  \"τS\" -> 0.040779763241   ,  \"τN\" -> 0.001074221992   ,  \"τC\" -> 0.001739718615   ,  \"κ0\" -> 0.000000003576   ,  \"mm1\" -> 0.000058137989   ,  \"mm2\" -> 0.020282386509   ,  \"mm3\" -> 0.045996711024   ,  \"T\" -> 0.620000000000   ,  \"B\" -> 10.000000000000   ,  \"θ\" -> 0.000000000000   ,  \"Reoff\" -> -1959183.673469394450   ,  \"Imoff\" -> 0.000000000000   ,  \"στ1\" -> 0.001449693425   ,  \"στS\" -> 0.000173563135   ,  \"στN\" -> 0.000045450535    |>   , \r\"IDS0433_220527_RAW_cal__sam_\" ->   <|    \"ζ\" -> 0.000000000000   ,  \"τ1\" -> 0.000000000000   ,  \"τS\" -> 0.000000000000   ,  \"τN\" -> 0.000000000000   ,  \"τC\" -> 0.000000000000   ,  \"κ0\" -> 0.000000000000   ,  \"mm1\" -> 0.000000000000   ,  \"mm2\" -> 0.000000000000   ,  \"mm3\" -> 0.000000000000   ,  \"T\" -> 0.620000000000   ,  \"B\" -> 10.000000000000   ,  \"θ\" -> 0.000000000000   ,  \"Reoff\" -> 0.000000000000   ,  \"Imoff\" -> 0.000000000000   ,  \"στ1\" -> 0.000000000000   ,  \"στS\" -> 0.000000000000   ,  \"στN\" -> 0.000000000000    |>   , \r\"IDS0434_220527_RAW_cal__ref_\" ->   <|    \"ζ\" -> 0.027519355554   ,  \"τ1\" -> 0.020590521074   ,  \"τS\" -> 0.048137141101   ,  \"τN\" -> 0.000693113139   ,  \"τC\" -> 0.001789335146   ,  \"κ0\" -> 0.000000004950   ,  \"mm1\" -> 0.000046291190   ,  \"mm2\" -> 0.020129239579   ,  \"mm3\" -> 0.052378356819   ,  \"T\" -> 0.820000000000   ,  \"B\" -> 10.000000000000   ,  \"θ\" -> 0.000000000000   ,  \"Reoff\" -> -1326530.612244904040   ,  \"Imoff\" -> 0.000000000000   ,  \"στ1\" -> 0.000620759114   ,  \"στS\" -> 0.000219619310   ,  \"στN\" -> 0.000010903062    |>   , \r\"IDS0434_220527_RAW_cal__sam_\" ->   <|    \"ζ\" -> 0.000000000000   ,  \"τ1\" -> 0.000000000000   ,  \"τS\" -> 0.000000000000   ,  \"τN\" -> 0.000000000000   ,  \"τC\" -> 0.000000000000   ,  \"κ0\" -> 0.000000000000   ,  \"mm1\" -> 0.000000000000   ,  \"mm2\" -> 0.000000000000   ,  \"mm3\" -> 0.000000000000   ,  \"T\" -> 0.820000000000   ,  \"B\" -> 10.000000000000   ,  \"θ\" -> 0.000000000000   ,  \"Reoff\" -> 0.000000000000   ,  \"Imoff\" -> 0.000000000000   ,  \"στ1\" -> 0.000000000000   ,  \"στS\" -> 0.000000000000   ,  \"στN\" -> 0.000000000000    |>   , \r\"IDS0435_220527_RAW_cal__ref_\" ->   <|    \"ζ\" -> 0.020842861739   ,  \"τ1\" -> 0.020135384195   ,  \"τS\" -> 0.018612634604   ,  \"τN\" -> 0.000305402785   ,  \"τC\" -> 0.002204389625   ,  \"κ0\" -> 0.000000007040   ,  \"mm1\" -> 0.000040405722   ,  \"mm2\" -> 0.018212466466   ,  \"mm3\" -> 0.023399245059   ,  \"T\" -> 1.120000000000   ,  \"B\" -> 10.000000000000   ,  \"θ\" -> 0.000000000000   ,  \"Reoff\" -> -693877.551020413636   ,  \"Imoff\" -> 0.000000000000   ,  \"στ1\" -> 0.001444867016   ,  \"στS\" -> 0.000117188914   ,  \"στN\" -> 0.000006503631    |>   , \r\"IDS0435_220527_RAW_cal__sam_\" ->   <|    \"ζ\" -> 0.000000000000   ,  \"τ1\" -> 0.000000000000   ,  \"τS\" -> 0.000000000000   ,  \"τN\" -> 0.000000000000   ,  \"τC\" -> 0.000000000000   ,  \"κ0\" -> 0.000000000000   ,  
